vi "Begin.vi"(8 "error in":errorcluster) -> (0 "error out":errorcluster)   [LabVIEW 2018]
doc: "Called before other user functions, this VI is expected to open initial I/O refnums, load in file data, and do all program initialization. Notice that the <B>error out</B> terminal is simply used for data flow. Wiring it to other structures or subVIs ensures that this VI runs first."
uses:
  <vilib>/Rock Robotics/WPI/DriverStation/WPI_DriverStationRobotMode2.ctl
  <vilib>/Rock Robotics/WPI/Joystick/WPI_JoystickDeviceEnum.ctl
  <vilib>/Rock Robotics/WPI/SerialPort/WPI_SerialPort.ctl
  Robot Global Data.vi
  <vilib>/Rock Robotics/Network Tables/NT Write String Array.vi
  <vilib>/Rock Robotics/WPI/ThirdParty/Phoenix-LabVIEW/Motor Controller/Controls/CTRE_Phoenix_MotorControl_NeutralMode.ctl
panel:
  out "error out 2":errorcluster
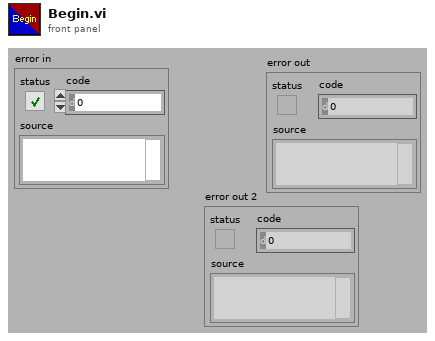
[diagram p1: front panel]
types:
  T1 = typedef "WPI_SerialPort.ctl" = enum16{"Onboard RS-232", "MXP TTL", "USB 1", "USB 2"}
  T2 = typedef "WPI_JoystickDeviceEnum.ctl" = enum16{"USB 0", "USB 1", "USB 2", "USB 3", "USB 4", "USB 5"}
  T3 = typedef "WPI_DriverStationRobotMode2.ctl" = enum16{"Autonomous Disabled", "Autonomous Enabled", "Teleop Disabled", "Teleop Enabled", "Disconnected", "Finish", "Test Disabled", "Test Enabled", "Emergency Stopped"}
  T4 = typedef "WPI_JoystickDevRef.ctl" = cluster{"Device":T2}
  T5 = typedef "WPI_SerialPortRef.ctl" = cluster{"DevStatus":errorcluster, "Serial Port Name":refnum<visa-resource-name>}
  T6 = cluster{"Master Left Motor":u8, "Left Motor":u8, "Master Right Motor":u8, "Right Motor":u8, "Master Butterfly Motor":i32, "Butterfly Motor":i32}
  T7 = typedef "WPI_MotorControlDeviceRef.ctl" = cluster{"DeviceStatus":errorcluster, "Type":T8, "PWM":cluster{"PWM Channel":T9, "DeadBand":T10}, "CAN":cluster{"Device Number":u8, "SetOutput VI Ref":variant, "GetOutput VI Ref":variant, "Enable VI Ref":variant, "Disable VI Ref":variant, "Data":variant}, "Invert":bool, "DIO PWM":cluster{"PWM \"Enable\" Channel":T9, "DIOChannel":T11, "PWM Rate":dbl}}
  T8 = typedef "WPI_MotorControlType.ctl" = enum16{"PWM", "CAN", "DIO PWM"}
  T9 = typedef "FPGA_DIOPWMChannel.ctl" = enum8{"PWM 0", "PWM 1", "PWM 2", "PWM 3", "PWM 4", "PWM 5", "PWM 6", "PWM 7", "PWM 8", "PWM 9", "PWM MXP 0", "PWM MXP 1", "PWM MXP 2", "PWM MXP 3", "PWM MXP 4", "PWM MXP 5", "PWM MXP 6", "PWM MXP 7", "PWM MXP 8", "PWM MXP 9", "Invalid"}
  T10 = typedef "WPI_PWMDeadband.ctl" = cluster{"Name":string, "maxPositivePwm":i32, "minPositivePwm":i32, "centerPwm":i32, "maxNegativePwm":i32, "minNegativePwm":i32, "angularRange":u16}
  T11 = typedef "FPGA_DIOChannel.ctl" = enum8{"DIO 0", "DIO 1", "DIO 2", "DIO 3", "DIO 4", "DIO 5", "DIO 6", "DIO 7", "DIO 8", "DIO 9", "DIO MXP 0", "DIO MXP 1", "DIO MXP 2", "DIO MXP 3", "DIO MXP 4", "DIO MXP 5", "DIO MXP 6", "DIO MXP 7", "DIO MXP 8", "DIO MXP 9", "DIO MXP 10", "DIO MXP 11", "DIO MXP 12", "DIO MXP 13", "DIO MXP 14", "DIO MXP 15", "SPI Port CS1", "SPI Port CS2", "SPI Port CS3", "SPI Port MISO", "SPI Port MOSI", "Invalid"}
  T12 = typedef "CTRE_Phoenix_MotorControl_NeutralMode.ctl" = enum8{"EEPROMSetting", "Override to Coast", "Override to Brake"}
  T13 = enum16{"FollowerType_PercentOutput", "FollowerType_AuxOutput1"}
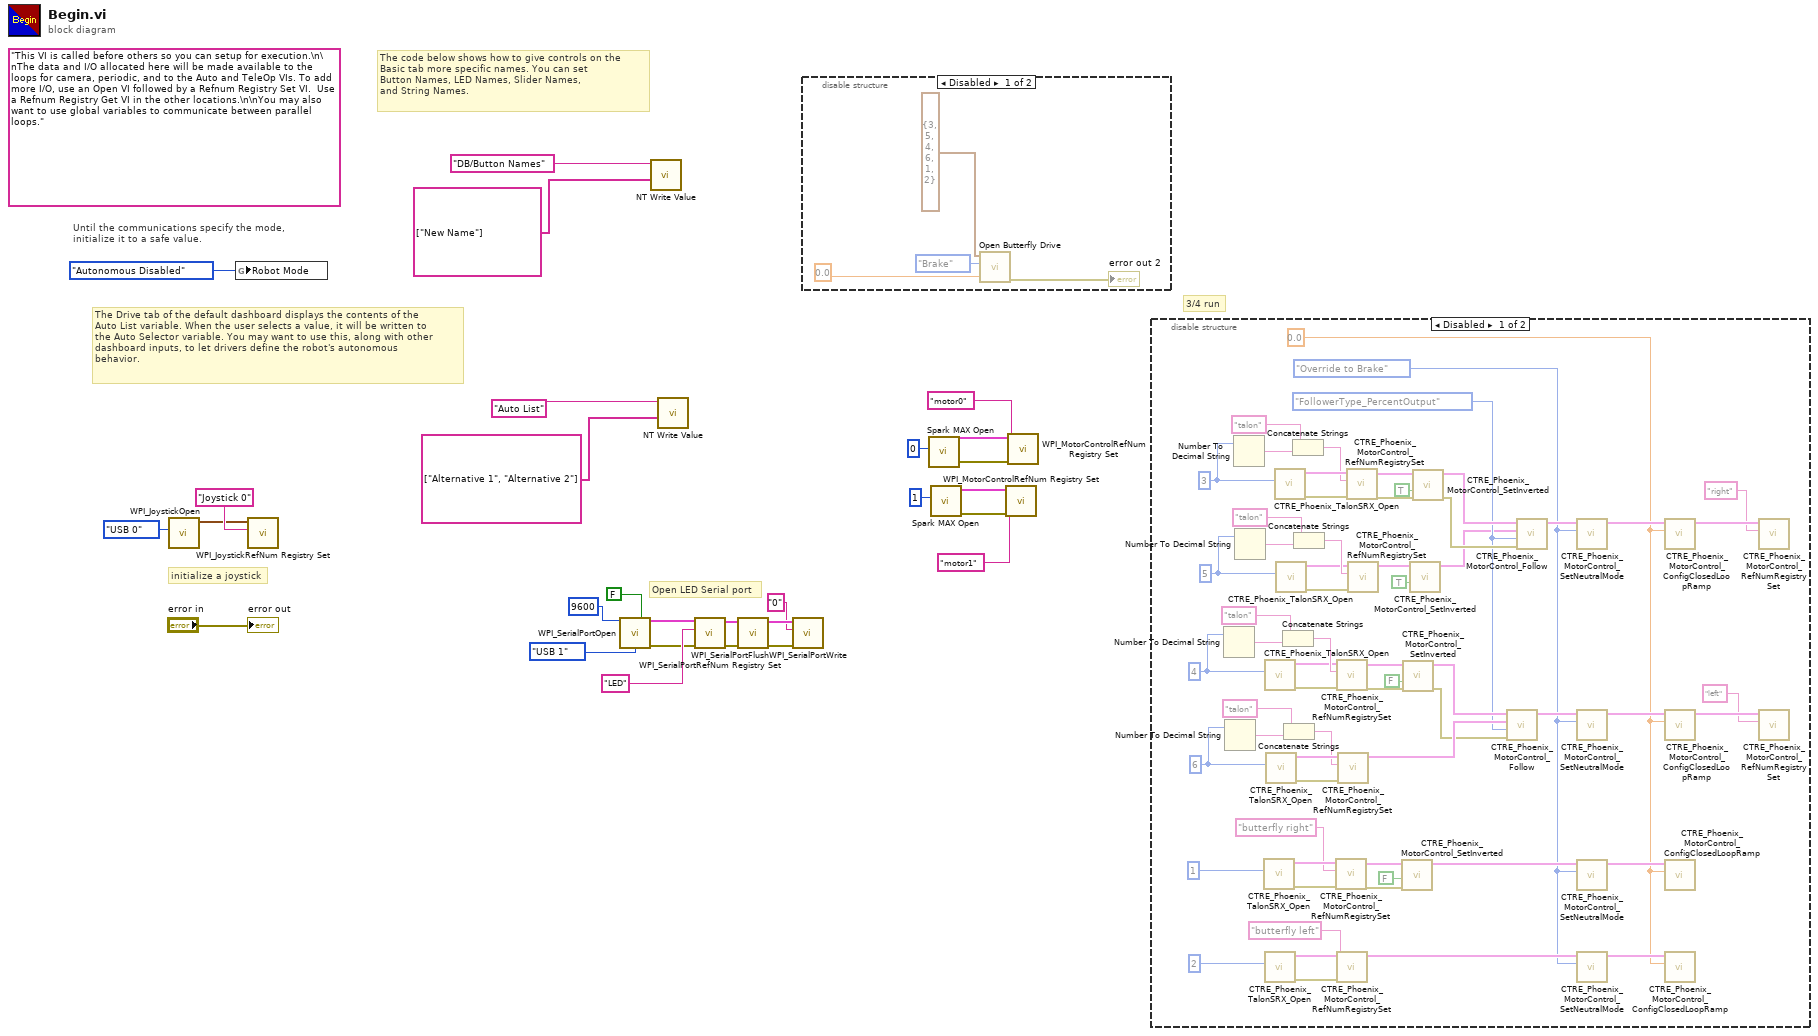
[diagram p0: block diagram]
diagram:
  (unwired) "This VI is called before others so you can setup for execution.\n\nThe data and I/O allocated here will be made available to the loops for camera, periodic, and to the Auto and TeleOp VIs. To add more I/O, use an Open VI followed by a Refnum Registry Set VI.  Use a Refnum Registry Get VI in the other locations.\n\nYou may also want to use global variables to communicate between parallel loops."
  # "Open LED Serial port"
  # "3/4 run"
  # "The Drive tab of the default dashboard displays the contents of the\nAuto List variable. When the user selects a value, it will be written to\nthe Auto Selector variable. You may want to use this, along with other\ndashboard inputs, to let drivers define the robot's autonomous\nbehavior."
  # "The code below shows how to give controls on the\nBasic tab more specific names. You can set\nButton Names, LED Names, Slider Names,\nand String Names."
  # "initialize a joystick"
  # "Until the communications specify the mode,\ninitialize it to a safe value."
  n1 = call <vilib>:"WPI_JoystickOpen.vi"("JoystickDevice"=WPI_JoystickDeviceEnum."USB 0") -> ("JoystickDevRef"=w26:T4)  [unwired: 10 in]
  n2 = global write "Robot Global Data.vi" "Robot Mode"(WPI_DriverStationRobotMode2."Autonomous Disabled" ("Robot Mode")) -> ()
  n3 = call <vilib>:"WPI_JoystickRefNum Registry Set.vi"("refnum name"="Joystick 0", "JoystickDevRef"=w26) -> ()  [unwired: 8 in, 2 out]
  n4 = call <vilib>:"WPI_SerialPortOpen.vi"("Baud Rate"=u32 9600, "Enable Termination Char? (T)"=FALSE, "Serial Port"=WPI_SerialPort."USB 1") -> ("SerialPortRef"=w17:T5, "error out"=w15:errorcluster)  [unwired: 11 in]
  n5 = call-poly <vilib>:"NT Write Value.vi"("String Array"=string[] ["New Name"], "Name"="DB/Button Names") -> ()  [unwired: 9 in, 1 out]
  n6 = call-poly <vilib>:"NT Write Value.vi"("String Array"=string[] ["Alternative 1", "Alternative 2"], "Name"="Auto List") -> ()  [unwired: 9 in, 1 out]
  n7 = call <vilib>:"WPI_SerialPortRefNum Registry Set.vi"("error in (no error)"=w15, "refnum name"="LED", "SerialPortRef"=w17) -> ("error out"=w11:errorcluster, "SerialPortRef"=w12:T5)  [unwired: 7 in]
  n8 = call <vilib>:"WPI_SerialPortFlush.vi"("error in (no error)"=w11, "SerialPortRef"=w12) -> ("error out"=w14:errorcluster, "SerialPortRef"=w13:T5)  [unwired: 8 in]
  n9 = call <vilib>:"WPI_SerialPortWrite.vi"("error in (no error)"=w14, "Buffer"="0", "SerialPortRef"=w13) -> ()  [unwired: 6 in, 3 out]
  n10 = disable-structure shown="Disabled" {
    frame Disabled {
      n11 = call "Open Butterfly Drive.vi"("secondsFromNeutralToFull"=0.0, "Brake/Coast"=enum16{"Coast", "Brake"}."Brake", "Cluster"=T6 {"Master Left Motor"=3, "Left Motor"=5, "Master Right Motor"=4, "Right Motor"=6, "Master Butterfly Motor"=1, "Butterfly Motor"=2}) -> ("error out"=→"error out 2":errorcluster)  [unwired: 8 in]
    }
    frame Enabled {
    }
  }
  n12 = call <vilib>:"Spark MAX Open.vi"("Device Number"=u8 0) -> ("error out"=w2:errorcluster, "MotorControlDeviceRef"=w3:T7)  [unwired: 9 in]
  n13 = call <vilib>:"Spark MAX Open.vi"("Device Number"=u8 1) -> ("error out"=w5:errorcluster, "MotorControlDeviceRef"=w6:T7)  [unwired: 9 in]
  n14 = call <vilib>:"WPI_MotorControlRefNum Registry Set.vi"("error in (no error)"=w5, "refnum name"="motor1", "MotorControlDevRef"=w6) -> ()  [unwired: 7 in, 2 out]
  n15 = call <vilib>:"WPI_MotorControlRefNum Registry Set.vi"("error in (no error)"=w2, "refnum name"="motor0", "MotorControlDevRef"=w3) -> ()  [unwired: 7 in, 2 out]
  n16 = disable-structure shown="Disabled" {
    frame Disabled {
      w37 = 0.0 ("secondsFromNeutralToFull")
      w36 = CTRE_Phoenix_MotorControl_NeutralMode."Override to Brake" ("Motor Control Neutral Mode")
      w48 = T13."FollowerType_PercentOutput" ("FollowerType")
      w70 = u8 6 ("Device Number")
      w63 = u8 4 ("Device Number")
      w84 = u8 5 ("Device Number")
      w91 = u8 3 ("Device Number")
      n17 = Number To Decimal String(number=w63) -> (decimal integer string=w64:string)  [unwired: 1 in]
      n18 = Number To Decimal String(number=w70) -> (decimal integer string=w69:string)  [unwired: 1 in]
      n19 = Number To Decimal String(number=w91) -> (decimal integer string=w90:string)  [unwired: 1 in]
      n20 = Number To Decimal String(number=w84) -> (decimal integer string=w85:string)  [unwired: 1 in]
      n21 = call <vilib>:"CTRE_Phoenix_TalonSRX_Open.vi"("Device Number"=u8 1) -> ("error out"=w56:errorcluster, "CAN Talon SRX Ref"=w55:T7)  [unwired: 9 in]
      n22 = call <vilib>:"CTRE_Phoenix_TalonSRX_Open.vi"("Device Number"=w63) -> ("error out"=w61:errorcluster, "CAN Talon SRX Ref"=w62:T7)  [unwired: 9 in]
      n23 = call <vilib>:"CTRE_Phoenix_TalonSRX_Open.vi"("Device Number"=u8 2) -> ("error out"=w51:errorcluster, "CAN Talon SRX Ref"=w52:T7)  [unwired: 9 in]
      n24 = call <vilib>:"CTRE_Phoenix_TalonSRX_Open.vi"("Device Number"=w70) -> ("error out"=w72:errorcluster, "CAN Talon SRX Ref"=w71:T7)  [unwired: 9 in]
      n25 = call <vilib>:"CTRE_Phoenix_TalonSRX_Open.vi"("Device Number"=w91) -> ("error out"=w93:errorcluster, "CAN Talon SRX Ref"=w92:T7)  [unwired: 9 in]
      n26 = call <vilib>:"CTRE_Phoenix_TalonSRX_Open.vi"("Device Number"=w84) -> ("error out"=w82:errorcluster, "CAN Talon SRX Ref"=w83:T7)  [unwired: 9 in]
      n27 = Concatenate Strings("talon" ("string"), w64) -> (w66:string)
      n28 = Concatenate Strings("talon" ("string"), w69) -> (w67:string)
      n29 = Concatenate Strings("talon" ("string"), w90) -> (w88:string)
      n30 = Concatenate Strings("talon" ("string"), w85) -> (w87:string)
      n31 = call <vilib>:"CTRE_Phoenix_MotorControl_RefNumRegistrySet.vi"("error in (no error)"=w56, "refnum name"="butterfly right", "PhoenixMotorControlDevRef"=w55) -> ("error out"=w49:errorcluster, "PhoenixMotorControlDevRef"=w50:T7)  [unwired: 7 in]
      n32 = call <vilib>:"CTRE_Phoenix_MotorControl_RefNumRegistrySet.vi"("error in (no error)"=w61, "refnum name"=w66, "PhoenixMotorControlDevRef"=w62) -> ("error out"=w74:errorcluster, "PhoenixMotorControlDevRef"=w73:T7)  [unwired: 7 in]
      n33 = call <vilib>:"CTRE_Phoenix_MotorControl_RefNumRegistrySet.vi"("error in (no error)"=w51, "refnum name"="butterfly left", "PhoenixMotorControlDevRef"=w52) -> ("PhoenixMotorControlDevRef"=w40:T7)  [unwired: 7 in, 1 out]
      n34 = call <vilib>:"CTRE_Phoenix_MotorControl_RefNumRegistrySet.vi"("error in (no error)"=w72, "refnum name"=w67, "PhoenixMotorControlDevRef"=w71) -> ("PhoenixMotorControlDevRef"=w77:T7)  [unwired: 7 in, 1 out]
      n35 = call <vilib>:"CTRE_Phoenix_MotorControl_RefNumRegistrySet.vi"("error in (no error)"=w93, "refnum name"=w88, "PhoenixMotorControlDevRef"=w92) -> ("error out"=w80:errorcluster, "PhoenixMotorControlDevRef"=w81:T7)  [unwired: 7 in]
      n36 = call <vilib>:"CTRE_Phoenix_MotorControl_RefNumRegistrySet.vi"("error in (no error)"=w82, "refnum name"=w87, "PhoenixMotorControlDevRef"=w83) -> ("PhoenixMotorControlDevRef"=w34:T7)  [unwired: 7 in, 1 out]
      n37 = call <vilib>:"CTRE_Phoenix_MotorControl_SetInverted.vi"("error in (no error)"=w49, "Invert?"=FALSE, "PhoenixMotorControlDevRef"=w50) -> ("PhoenixMotorControlDevRef"=w41:T7)  [unwired: 7 in, 1 out]
      n38 = call <vilib>:"CTRE_Phoenix_MotorControl_SetInverted.vi"("error in (no error)"=w74, "Invert?"=FALSE, "PhoenixMotorControlDevRef"=w73) -> ("error out"=w75:errorcluster, "PhoenixMotorControlDevRef"=w76:T7)  [unwired: 7 in]
      n39 = call <vilib>:"CTRE_Phoenix_MotorControl_SetInverted.vi"("Invert?"=TRUE, "PhoenixMotorControlDevRef"=w34) -> ("PhoenixMotorControlDevRef"=w33:T7)  [unwired: 8 in, 1 out]
      n40 = call <vilib>:"CTRE_Phoenix_MotorControl_SetInverted.vi"("error in (no error)"=w80, "Invert?"=TRUE, "PhoenixMotorControlDevRef"=w81) -> ("error out"=w79:errorcluster, "PhoenixMotorControlDevRef"=w78:T7)  [unwired: 7 in]
      n41 = call <vilib>:"CTRE_Phoenix_MotorControl_Follow.vi"("error in (no error)"=w75, "FollowerType"=w48, "Master Controller to Follow"=w77, "PhoenixMotorControlDevRef"=w76) -> ("PhoenixMotorControlDevRef"=w59:T7)  [unwired: 6 in, 1 out]
      n42 = call <vilib>:"CTRE_Phoenix_MotorControl_Follow.vi"("error in (no error)"=w79, "FollowerType"=w48, "Master Controller to Follow"=w33, "PhoenixMotorControlDevRef"=w78) -> ("PhoenixMotorControlDevRef"=w95:T7)  [unwired: 6 in, 1 out]
      n43 = call <vilib>:"CTRE_Phoenix_MotorControl_SetNeutralMode.vi"("Motor Control Neutral Mode"=w36, "PhoenixMotorControlDevRef"=w95) -> ("PhoenixMotorControlDevRef"=w94:T7)  [unwired: 8 in, 1 out]
      n44 = call <vilib>:"CTRE_Phoenix_MotorControl_SetNeutralMode.vi"("Motor Control Neutral Mode"=w36, "PhoenixMotorControlDevRef"=w59) -> ("PhoenixMotorControlDevRef"=w60:T7)  [unwired: 8 in, 1 out]
      n45 = call <vilib>:"CTRE_Phoenix_MotorControl_SetNeutralMode.vi"("Motor Control Neutral Mode"=w36, "PhoenixMotorControlDevRef"=w41) -> ("PhoenixMotorControlDevRef"=w38:T7)  [unwired: 8 in, 1 out]
      n46 = call <vilib>:"CTRE_Phoenix_MotorControl_SetNeutralMode.vi"("Motor Control Neutral Mode"=w36, "PhoenixMotorControlDevRef"=w40) -> ("PhoenixMotorControlDevRef"=w39:T7)  [unwired: 8 in, 1 out]
      n47 = call <vilib>:"CTRE_Phoenix_MotorControl_ConfigClosedLoopRamp.vi"("secondsFromNeutralToFull"=w37, "PhoenixMotorControlDevRef"=w94) -> ("PhoenixMotorControlDevRef"=w47:T7)  [unwired: 8 in, 1 out]
      n48 = call <vilib>:"CTRE_Phoenix_MotorControl_ConfigClosedLoopRamp.vi"("secondsFromNeutralToFull"=w37, "PhoenixMotorControlDevRef"=w60) -> ("PhoenixMotorControlDevRef"=w46:T7)  [unwired: 8 in, 1 out]
      n49 = call <vilib>:"CTRE_Phoenix_MotorControl_ConfigClosedLoopRamp.vi"("secondsFromNeutralToFull"=w37, "PhoenixMotorControlDevRef"=w38) -> ()  [unwired: 8 in, 2 out]
      n50 = call <vilib>:"CTRE_Phoenix_MotorControl_ConfigClosedLoopRamp.vi"("secondsFromNeutralToFull"=w37, "PhoenixMotorControlDevRef"=w39) -> ()  [unwired: 8 in, 2 out]
      n51 = call <vilib>:"CTRE_Phoenix_MotorControl_RefNumRegistrySet.vi"("refnum name"="right", "PhoenixMotorControlDevRef"=w47) -> ()  [unwired: 8 in, 2 out]
      n52 = call <vilib>:"CTRE_Phoenix_MotorControl_RefNumRegistrySet.vi"("refnum name"="left", "PhoenixMotorControlDevRef"=w46) -> ()  [unwired: 8 in, 2 out]
    }
    frame Enabled {
    }
  }
  "error out" <- "error in"
